vi "PC_Controller.vi"() -> ()   [LabVIEW 2017]
uses:
  <vilib>/NI/STM/NI STM.lvlib
  Components/TypeDefs/UI StateDef_Enum.ctl
  <vilib>/NI/STM/TCP/TCP Read Options.ctl
  <vilib>/NI/STM/TCP/Read Meta Data (TCP Ref).vi
  <vilib>/NI/STM/TCP/Read Message (TCP).vi
  <vilib>/Utility/sysdir.llb/System Directory Type.ctl
  <vilib>/Utility/file.llb/Write Delimited Spreadsheet (DBL).vi
  <vilib>/NI/STM/TCP/Get Connection Reference (TCP).vi
panel:
  in  "Save charts":bool
  out "RT loop time [sec]":dbl
  in  "Pause Charts":bool
  out "# of elements \nremoved":i32
  in  "Clear charts":bool
  out "Raw Measurements":dbl[][](graph)
  out "Status....":string
  out "Loop time (sec)":dbl
  in  "Stop Button":bool
  out "Coil voltages":dbl[][](graph)
  out "Control Efforts":dbl[][](graph)
  out "Coordinate Transformed Measurements":dbl[][](graph)
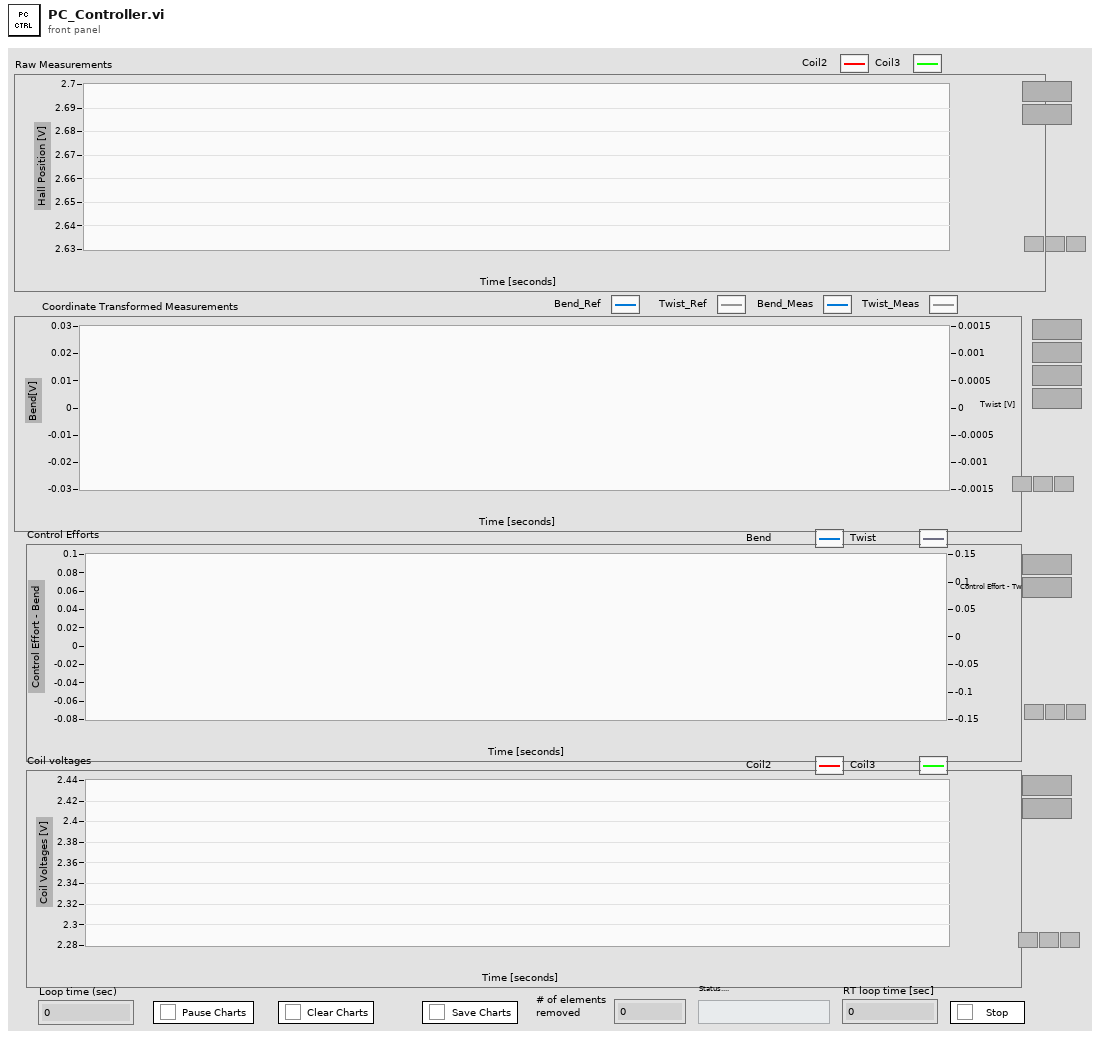
[diagram p1: front panel]
types:
  T1 = typedef "NI STM.lvlib/TCP Read Options.ctl" = cluster{"ignore timeout error":bool, "timeout ms (1000)":i32}
  T2 = typedef "UI StateDef_Enum.ctl" = enum16{"Initialize", "Wait", "Update AO", "Stop", "Set 0 level Ch", "Clear Charts", "Pause Charts", "Save charts"}
  T3 = typedef "NI STM.lvlib/TCP Connection Info.ctl" = cluster{"connection ID":refnum<k5>, "meta data":T4[]}
  T4 = typedef "NI STM.lvlib/MetaDataElement.ctl" = string
  T5 = typedef "System Directory Type.ctl" = i32
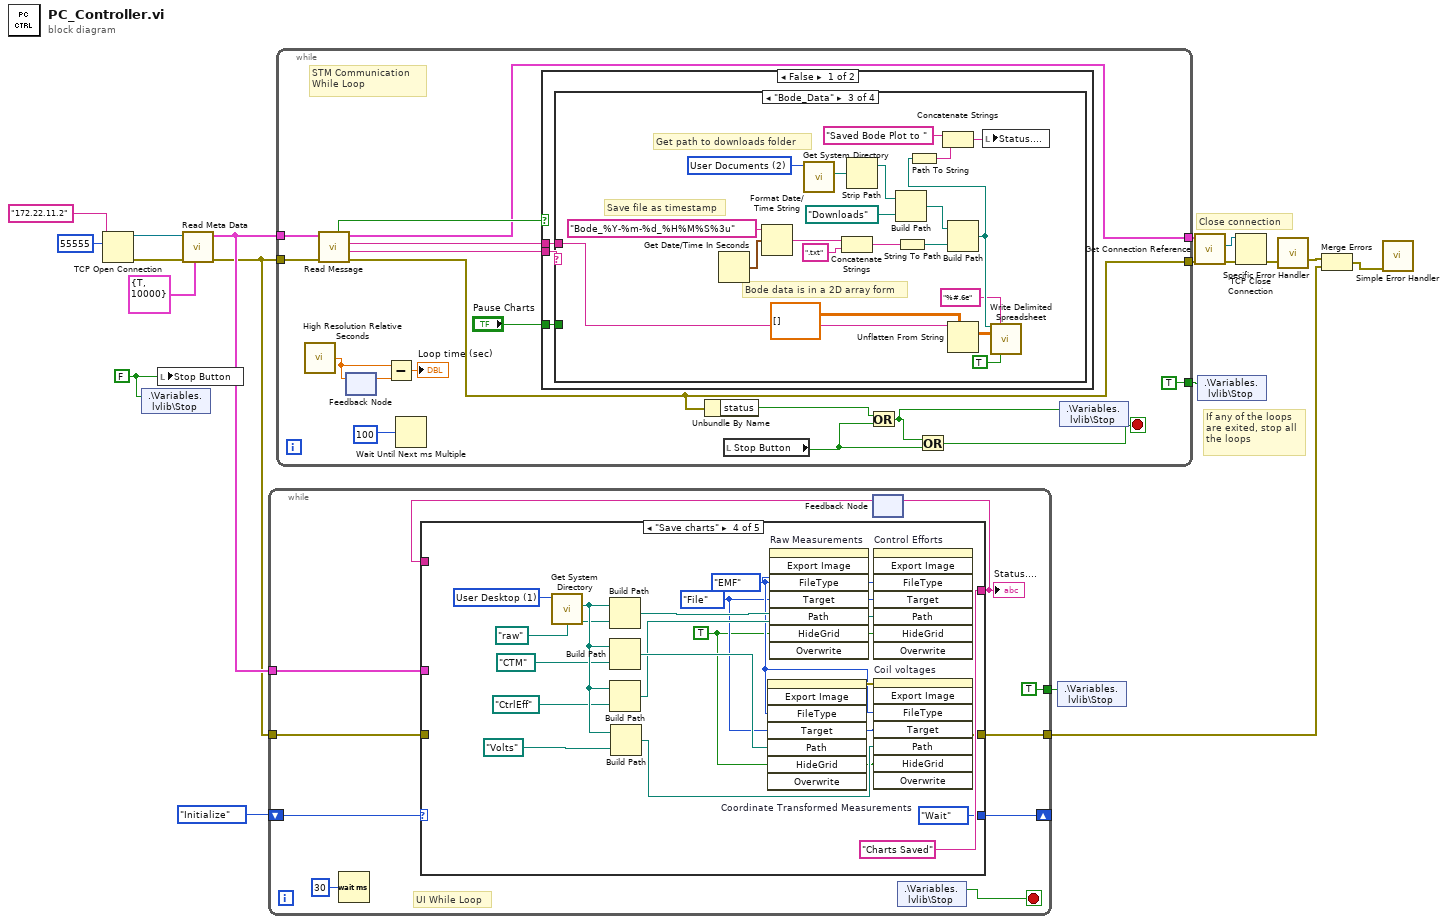
[diagram p0: block diagram]
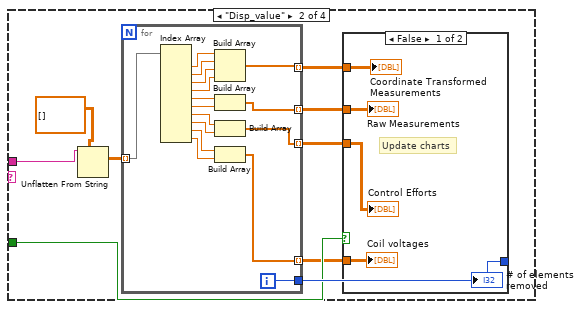
[diagram p3: hidden frame]
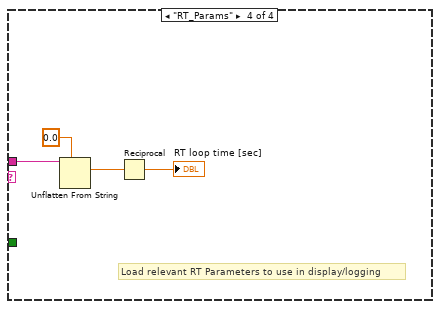
[diagram p5: hidden frame]
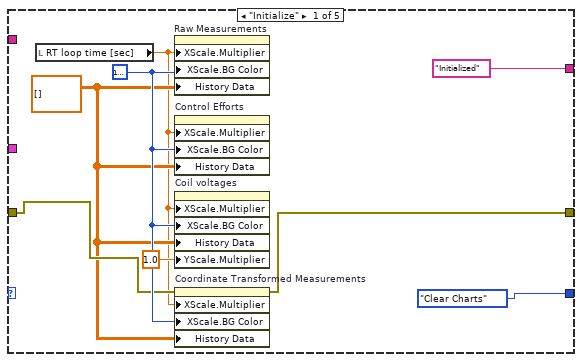
[diagram p7: hidden frame]
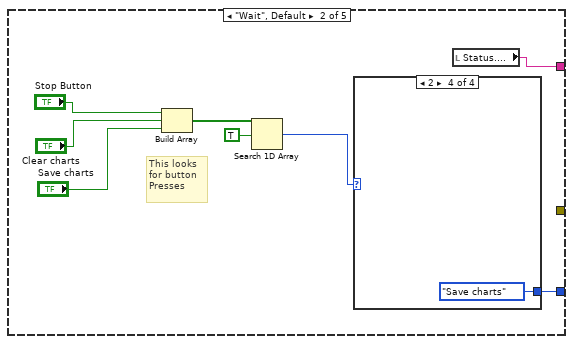
[diagram p8: hidden frame]
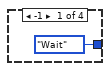
[diagram p9: hidden frame]
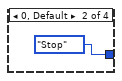
[diagram p10: hidden frame]
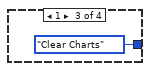
[diagram p11: hidden frame]
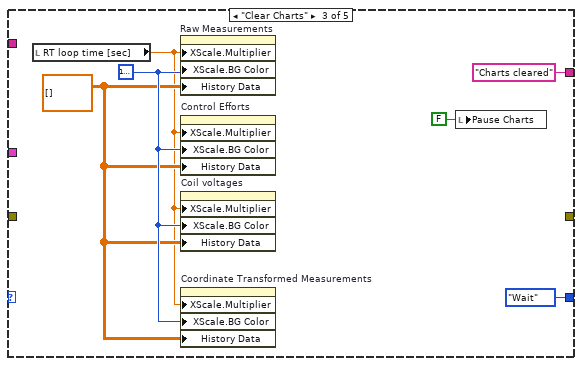
[diagram p12: hidden frame]
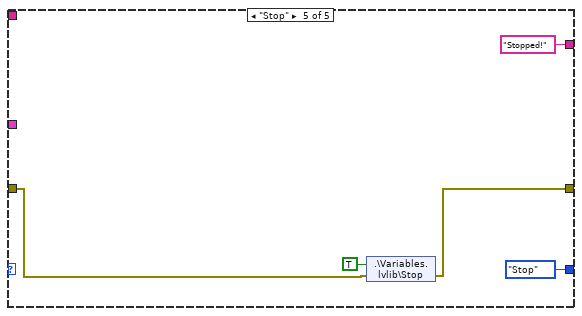
[diagram p13: hidden frame]
diagram:
  w10 = FALSE ("System Stop Button")
  # "Close connection"
  # "If any of the loops\nare exited, stop all \nthe loops"
  n1 = TCP Open Connection(address="172.22.11.2", remote port or service name=u16 55555) -> (connection ID=w17:refnum<k5>, error out=w16:errorcluster)  [unwired: 3 in]
  n2 = shared-variable ".\\Variables.lvlib\\Stop"(w10) -> ()  [unwired: 1 in, 1 out]
  n3 = local write "Stop Button"(w10) -> ()
  n4 = call-poly <vilib>:"Read Meta Data.vi"("options"=T1 {"ignore timeout error"=TRUE, "timeout ms (1000)"=10000}, "error in"=w16, "connection ID"=w17) -> ("error out"=w7:errorcluster, "connection info out"=w8:T3)  [unwired: 6 in, 1 out]
  n5 = while {
    shift-right: [w25] -> _
    shift-left: UI_StateDef_Enum."Initialize" ("UI StateDef_Enum") -> [w29]
    tunnel: w8 -> [w27]
    tunnel: w7 -> [w22]
    tunnel: [w21] -> w5
    tunnel: [TRUE ("Stop")] -> w2
    stop <- w28 stop-if-true
    # "UI While Loop"
    n6 = Wait (ms)(milliseconds to wait=u32 30) -> ()  [unwired: 1 out]
    n7 = feedback #1() -> (w23:string)  [unwired: 1 in]
    n8 = case shown="\"Save charts\"" w29 {
      tunnel: [UI_StateDef_Enum."Clear Charts" ("UI StateDef_Enum") w41 UI_StateDef_Enum."Wait" ("UI StateDef_Enum") UI_StateDef_Enum."Wait" ("UI StateDef_Enum") UI_StateDef_Enum."Stop" ("UI StateDef_Enum")] -> w25
      tunnel: ["Initialized" ("Status....") w39 "Charts cleared" ("Status....") "Charts Saved" ("Status....") "Stopped!" ("Status....")] -> w24
      tunnel: w27 -> [_ _ _ _ _]
      tunnel: w23 -> [_ _ _ _ _]
      tunnel: w22 -> [w34 _ _ _ w73]
      tunnel: [w33 _ _ w60 w74] -> w21
      frame "Initialize" {
        w31 = dbl[][] [] ("History Data")
        w35 = u32 16777216 ("X Scale.Marker Colors:BG Color")
        n9 = local read "RT loop time [sec]"() -> (w30:dbl)
        n10 = property on="Raw Measurements" class="WFChart (strict)"("XScale.Multiplier"=w30, "XScale.BG Color"=w35, "History Data"=w31) -> ()  [unwired: 2 in, 2 out]
        n11 = property on="Control Efforts" class="WFChart (strict)"("XScale.Multiplier"=w30, "XScale.BG Color"=w35, "History Data"=w31) -> ()  [unwired: 2 in, 2 out]
        n12 = property on="Coil voltages" class="WFChart (strict)"("XScale.Multiplier"=w30, "XScale.BG Color"=w35, "History Data"=w31, "YScale.Multiplier"=1.0 ("Y Scale.Offset and Multiplier:Multiplier")) -> ()  [unwired: 2 in, 2 out]
        n13 = property on="Coordinate Transformed Measurements" class="WFChart (strict)"(error in=w34, "XScale.Multiplier"=w30, "XScale.BG Color"=w35, "History Data"=w31) -> (error out=w33:errorcluster)  [unwired: 1 in, 1 out]
      }
      frame "Wait", Default {
        # "This looks \nfor button \nPresses"
        n14 = Build Array "Build Array"("Stop Button", "Clear charts", "Save charts") -> (w45:bool[])
        n15 = Search 1D Array(1D array=w45, element=TRUE) -> (index of element=w44:i32)  [unwired: 1 in]
        n16 = case shown="2" w44 {
          tunnel: [UI_StateDef_Enum."Wait" ("UI StateDef_Enum") UI_StateDef_Enum."Stop" ("UI StateDef_Enum") UI_StateDef_Enum."Clear Charts" ("UI StateDef_Enum") UI_StateDef_Enum."Save charts" ("UI StateDef_Enum")] -> w41
          frame -1 {
          }
          frame 0, Default {
          }
          frame 1 {
          }
          frame 2 {
          }
        }
        n17 = local read "Status...."() -> (w39:string)
      }
      frame "Clear Charts" {
        w52 = dbl[][] [] ("History Data")
        w55 = u32 16777216 ("X Scale.Marker Colors:BG Color")
        n18 = local read "RT loop time [sec]"() -> (w50:dbl)
        n19 = property on="Raw Measurements" class="WFChart (strict)"("XScale.Multiplier"=w50, "XScale.BG Color"=w55, "History Data"=w52) -> ()  [unwired: 2 in, 2 out]
        n20 = property on="Control Efforts" class="WFChart (strict)"("XScale.Multiplier"=w50, "XScale.BG Color"=w55, "History Data"=w52) -> ()  [unwired: 2 in, 2 out]
        n21 = property on="Coil voltages" class="WFChart (strict)"("XScale.Multiplier"=w50, "XScale.BG Color"=w55, "History Data"=w52) -> ()  [unwired: 2 in, 2 out]
        n22 = property on="Coordinate Transformed Measurements" class="WFChart (strict)"("XScale.Multiplier"=w50, "XScale.BG Color"=w55, "History Data"=w52) -> ()  [unwired: 2 in, 2 out]
        n23 = local write "Pause Charts"(FALSE ("Pause Charts")) -> ()
      }
      frame "Save charts" {
        w70 = T5 1 items=["User Home"=0, "User Desktop"=1, "User Documents"=2, "User Application Data"=3, "User Preferences"=4, "User Temporary"=5, "Public Documents"=6, "Public Application Data"=7, "Public Preferences"=8, "Public Cache"=13, "System Core Libraries"=9, "System Installed Libraries"=10, "Application Files"=11, "Boot Volume Root"=12] ("system directory type")
        w56 = TRUE ("Hide Grid")
        w57 = enum32{"File", "Clipboard"}."File" ("Target")
        w58 = enum32{"BMP", "EPS", "EMF", "PICT"}."EMF" ("File Type")
        n24 = call <vilib>:"Get System Directory.vi"("system directory type"=w70) -> ("system directory"=w69:path)  [unwired: 10 in]
        n25 = Build Path(base path=w69, name or relative path=path "raw") -> (appended path=w64:path)
        n26 = Build Path(base path=w69, name or relative path=path "CTM") -> (appended path=w63:path)
        n27 = Build Path(base path=w69, name or relative path=path "CtrlEff") -> (appended path=w62:path)
        n28 = Build Path(base path=w69, name or relative path=path "Volts") -> (appended path=w61:path)
        n29 = invoke on="Coordinate Transformed Measurements" class="WFChart (strict)" method="Export Image"("FileType"=w58, "Target"=w57, "Path"=w63, "HideGrid"=w56) -> (error out=w71:errorcluster)  [unwired: 4 in, 7 out]
        n30 = invoke on="Raw Measurements" class="WFChart (strict)" method="Export Image"("FileType"=w58, "Target"=w57, "Path"=w64, "HideGrid"=w56) -> ()  [unwired: 4 in, 8 out]
        n31 = invoke on="Control Efforts" class="WFChart (strict)" method="Export Image"("FileType"=w58, "Target"=w57, "Path"=w62, "HideGrid"=w56) -> ()  [unwired: 4 in, 8 out]
        n32 = invoke on="Coil voltages" class="WFChart (strict)" method="Export Image"(error in=w71, "FileType"=w58, "Target"=w57, "Path"=w61, "HideGrid"=w56) -> (error out=w60:errorcluster)  [unwired: 3 in, 7 out]
      }
      frame "Stop" {
        n33 = shared-variable ".\\Variables.lvlib\\Stop"(TRUE ("Stop"), error in=w73) -> (error out=w74:errorcluster)
      }
    }
    "Status...." <- w24
    n34 = feedback-in #1(w24) -> ()
    n35 = shared-variable ".\\Variables.lvlib\\Stop"() -> (w28:bool)  [unwired: 1 in, 1 out]
  }
  n36 = while {
    tunnel: w8 -> [w94]
    tunnel: w7 -> [w93]
    tunnel: [w91] -> w12
    tunnel: [w90] -> w11
    tunnel: [TRUE ("Stop")] -> w3
    stop <- w84 stop-if-true
    # "STM Communication\nWhile Loop"
    n37 = call <vilib>:"High Resolution Relative Seconds.vi"() -> ("relative seconds"=w86:dbl)
    n38 = call-poly <vilib>:"Read Message.vi"("error in"=w93, "connection info in"=w94) -> ("error out"=w90:errorcluster, "name"=w89:T4, "data string"=w88:string, "connection info out"=w91:T3, "timed out?"=w92:bool)  [unwired: 4 in, 1 out]
    n39 = feedback-in #2(w86) -> ()
    n40 = feedback #2() -> (w87:dbl)  [unwired: 1 in]
    n41 = Subtract(x=w86, y=w87) -> (x-y=→"Loop time (sec)":dbl)
    n42 = Wait Until Next ms Multiple(millisecond multiple=u32 100 ("Period")) -> ()  [unwired: 1 out]
    n43 = case shown="False" w92 {
      tunnel: w89 -> [w97 _]
      tunnel: w88 -> [w96 _]
      tunnel: "Pause Charts" -> [w95 _]
      frame False {
        n44 = case shown="\"Bode_Data\"" w97 {
          tunnel: w96 -> [_ w106 w131 w151]
          tunnel: w95 -> [_ w102 _ _]
          frame Default {
          }
          frame "Disp_value" {
            n45 = Unflatten From String(type=dbl[][] [], binary string=w106) -> (value=w104:dbl[][])  [unwired: 3 in, 2 out]
            n46 = for {
              tunnel: w104 -> [w126] mode=indexing
              tunnel: [w127] -> w103
              tunnel: [w125] -> w101 mode=indexing
              tunnel: [w118] -> w100 mode=indexing
              tunnel: [w115] -> w99 mode=indexing
              tunnel: [w112] -> w98 mode=indexing
              i -> [w127]
              n47 = Index Array(array=w126) -> (element #1=w124:dbl, element #2=w123:dbl, element #3=w122:dbl, element #4=w121:dbl, element #5=w120:dbl, element #6=w119:dbl, element #7=w117:dbl, element #8=w116:dbl, element #9=w114:dbl, element #10=w113:dbl)  [unwired: 10 in]
              n48 = Build Array(w124, w123, w122, w121) -> (w125:dbl[])
              n49 = Build Array(w120, w119) -> (w118:dbl[])
              n50 = Build Array(w117, w116) -> (w115:dbl[])
              n51 = Build Array(w114, w113) -> (w112:dbl[])
            }
            n52 = case shown="False" w102 {
              tunnel: w103 -> [w111 _]
              tunnel: w101 -> [w110 _]
              tunnel: w100 -> [w109 _]
              tunnel: w99 -> [w108 _]
              tunnel: w98 -> [w107 _]
              frame False {
                # "Update charts"
                "Raw Measurements" <- w109
                "Coordinate Transformed Measurements" <- w110
                "Control Efforts" <- w108
                "Coil voltages" <- w107
                "# of elements \nremoved" <- w111
              }
              frame True {
              }
            }
          }
          frame "Bode_Data" {
            w145 = T5 2 items=["User Home"=0, "User Desktop"=1, "User Documents"=2, "User Application Data"=3, "User Preferences"=4, "User Temporary"=5, "Public Documents"=6, "Public Application Data"=7, "Public Preferences"=8, "Public Cache"=13, "System Core Libraries"=9, "System Installed Libraries"=10, "Application Files"=11, "Boot Volume Root"=12] ("system directory type")
            # "Save file as timestamp"
            # "Get path to downloads folder"
            # "Bode data is in a 2D array form"
            n53 = Get Date/Time In Seconds() -> (seconds since 1Jan1904=w142:timestamp)
            n54 = Format Date/Time String(time format string (%c)="Bode_%Y-%m-%d_%H%M%S%3u", seconds (now)=w142) -> (date/time string=w137:string)  [unwired: 1 in]
            n55 = call <vilib>:"Get System Directory.vi"("system directory type"=w145) -> ("system directory"=w144:path)  [unwired: 10 in]
            n56 = Concatenate Strings(w137, ".txt" ("string")) -> (w138:string)
            n57 = Strip Path(path=w144) -> (stripped path=w143:path)  [unwired: 1 out]
            n58 = Build Path(base path=w143, name or relative path=path "Downloads" ("file path (dialog if empty)")) -> (appended path=w139:path)
            n59 = String To Path(string=w138) -> (path=w140:path)
            n60 = Build Path(base path=w139, name or relative path=w140) -> (appended path=w132:path)
            n61 = Path To String(path=w132) -> (string=w133:string)
            n62 = Concatenate Strings("Saved Bode Plot to " ("string"), w133) -> (w129:string)
            n63 = Unflatten From String(type=dbl[][] [], binary string=w131) -> (value=w135:dbl[][])  [unwired: 3 in, 2 out]
            n64 = local write "Status...."(w129) -> ()
            n65 = call-poly <vilib>:"Write Delimited Spreadsheet.vi"("file path (dialog if empty)"=w132, "format (%.3f)"="%#.6e", "2D data"=w135, "transpose? (no:F)"=TRUE) -> ()  [unwired: 10 in, 2 out]
          }
          frame "RT_Params" {
            # "Load relevant RT Parameters to use in display/logging"
            n66 = Unflatten From String(type=0.0, binary string=w151) -> (value=w149:dbl)  [unwired: 3 in, 2 out]
            n67 = Reciprocal(x=w149) -> (1/x=→"RT loop time [sec]":dbl)
          }
        }
      }
      frame True {
      }
    }
    n68 = Unbundle By Name(w90) -> ("status"=w82:bool)
    n69 = local read "Stop Button"() -> (w83:bool)
    n70 = Or(x=w82, y=w83) -> (x .or. y?=w81:bool)
    n71 = Or(x=w81, y=w83) -> (x .or. y?=w84:bool)
    n72 = shared-variable ".\\Variables.lvlib\\Stop"(w81) -> ()  [unwired: 1 in, 1 out]
  }
  n73 = shared-variable ".\\Variables.lvlib\\Stop"(w2) -> ()  [unwired: 1 in, 1 out]
  n74 = call-poly <vilib>:"Get Connection Reference.vi"("error in"=w11, "connection info in"=w12) -> ("error out"=w15:errorcluster, "connection ID out"=w14:refnum<k5>)  [unwired: 7 in, 1 out]
  n75 = shared-variable ".\\Variables.lvlib\\Stop"(w3) -> ()  [unwired: 1 in, 1 out]
  n76 = TCP Close Connection(connection ID=w14, error in (no error)=w15) -> (error out=w13:errorcluster)  [unwired: 1 in, 1 out]
  n77 = call "Specific Error Handler"("Error to Check"=w13) -> ("error out"=w4:errorcluster)  [unwired: 11 in, 3 out]
  n78 = Merge Errors(w4, w5) -> (w6:errorcluster)
  n79 = call <vilib>:"Simple Error Handler.vi"("error in (no error)"=w6) -> ()  [unwired: 4 in, 5 out]
